vi "Begin.vi"() -> (0 "error out":errorcluster)   [LabVIEW 2013]
doc: "Called before other user functions, this VI is expected to open initial I/O refnums, load in file data, and do all program initialization. Notice that the <B>error out</B> terminal is simply used for data flow. Wiring it to other structures or subVIs ensures that this VI runs first."
uses:
  <vilib>/Rock Robotics/WPI/DriverStation/WPI_DriverStationRobotMode2.ctl
  <vilib>/Rock Robotics/WPI/Joystick/WPI_JoystickDeviceEnum.ctl
  <vilib>/Rock Robotics/SystemInterfaces/DIO/FPGA_DIOPWMChannel.ctl
  <vilib>/Rock Robotics/SystemInterfaces/Typedef/FPGA_TypedefDigitalModule.ctl
  <vilib>/Rock Robotics/WPI/SafetyOutput/WPI_SafetyOutputConfigMenu.ctl
  Robot Global Data.vi
  Device Refrences.vi
  <vilib>/Rock Robotics/WPI/RobotDrive/WPI_RobotDriveOpen2MotorWithJaguar.vi
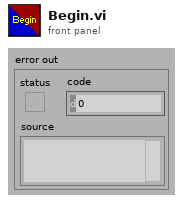
[diagram p1: front panel]
types:
  T1 = typedef "WPI_JoystickDeviceEnum.ctl" = enum16{"USB 1", "USB 2", "USB 3", "USB 4", "Kinect 1", "Kinect 2"}
  T2 = enum16{"1 3-axis Joystick", "2 2-axis Joysticks"}
  T3 = typedef "WPI_DriverStationRobotMode2.ctl" = enum16{"Autonomous Disabled", "Autonomous Enabled", "Teleop Disabled", "Teleop Enabled", "Timeout", "Finish", "Test Disabled", "Test Enabled"}
  T4 = typedef "WPI_JoystickDevRef.ctl" = cluster{"Device":T1}
  T5 = enum16{"Simulator Robot", "Alpinista", "2014 Robot"}
  T6 = typedef "FPGA_TypedefDigitalModule.ctl" = enum16{"Digital Module 1", "Digital Module 2"}
  T7 = typedef "FPGA_DIOPWMChannel.ctl" = enum8{"PWM 1", "PWM 2", "PWM 3", "PWM 4", "PWM 5", "PWM 6", "PWM 7", "PWM 8", "PWM 9", "PWM 10", "Invalid"}
  T8 = typedef "WPI_ServoDeviceRef.ctl" = cluster{"DeviceStatus":errorcluster, "Digital Module":T6, "PWM Channel":T7, "DeadBand":T9}
  T9 = typedef "WPI_PWMDeadband.ctl" = cluster{"Name":string, "maxPositivePwm":i32, "minPositivePwm":i32, "centerPwm":i32, "maxNegativePwm":i32, "minNegativePwm":i32, "angularRange":u16}
  T10 = typedef "WPI_SafetyOutputConfigMenu.ctl" = enum16{"Enable", "Disable"}
  T11 = typedef "WPI_RobotDriveDevRef.ctl" = cluster{"DevStatus":errorcluster, "Motors[]":T12[], "Square Inputs":bool, "Max Output":dbl, "Isochronous":bool}
  T12 = typedef "WPI_MotorControlDeviceRef.ctl" = cluster{"DeviceStatus":errorcluster, "Type":enum16{"PWM", "CAN"}, "PWM":cluster{"Digital Module":T6, "PWM Channel":T7, "DeadBand":T9}, "CAN":cluster{"Device Number":u8, "Control Mode":T13, "Semaphore":T14, "Max Vout":dbl}, "Invert":bool, "TransformRef":T15, "InvTransformRef":T15}
  T13 = typedef "WPI_CANJaguar_ControlMode.ctl" = enum8{"Percent VBus", "Current", "Speed", "Position", "Voltage"}
  T14 = typedef "Semaphore RefNum" = refnum<k1>
  T15 = typedef "WPI_PWMTransform_ConPane.ctl" = refnum<vi>
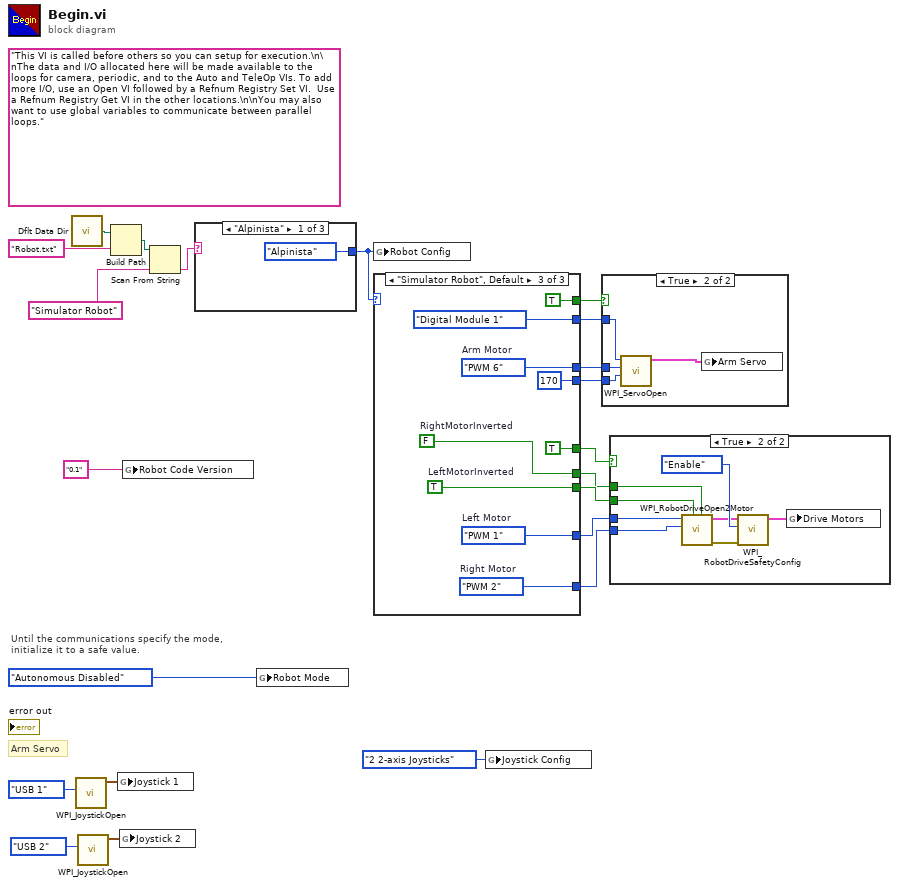
[diagram p0: block diagram]
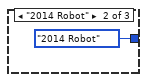
[diagram p4: hidden frame]
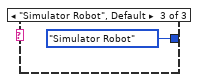
[diagram p5: hidden frame]
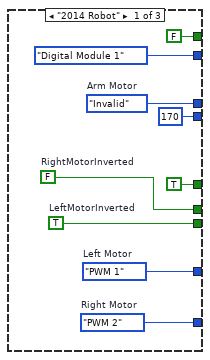
[diagram p6: hidden frame]
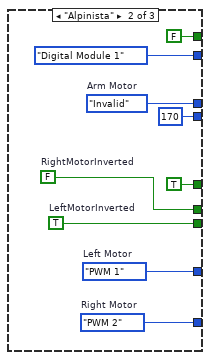
[diagram p7: hidden frame]
diagram:
  (unwired) "This VI is called before others so you can setup for execution.\n\nThe data and I/O allocated here will be made available to the loops for camera, periodic, and to the Auto and TeleOp VIs. To add more I/O, use an Open VI followed by a Refnum Registry Set VI.  Use a Refnum Registry Get VI in the other locations.\n\nYou may also want to use global variables to communicate between parallel loops."
  # "Arm Servo"
  # "Until the communications specify the mode,\ninitialize it to a safe value."
  n1 = call <vilib>:"Dflt Data Dir.vi"() -> ("App:Default Data Directory"=w11:path)
  n2 = call <vilib>:"WPI_JoystickOpen.vi"("JoystickDevice"=WPI_JoystickDeviceEnum."USB 1") -> ("JoystickDevRef"=w20:T4)  [unwired: 10 in]
  n3 = call <vilib>:"WPI_JoystickOpen.vi"("JoystickDevice"=WPI_JoystickDeviceEnum."USB 2") -> ("JoystickDevRef"=w2:T4)  [unwired: 10 in]
  n4 = Build Path(base path=w11, name or relative path="Robot.txt") -> (appended path=w5:path)
  n5 = global write "Device Refrences.vi" "Joystick 1"(w20) -> ()
  n6 = global write "Device Refrences.vi" "Joystick 2"(w2) -> ()
  n7 = global write "Robot Global Data.vi" "Robot Code Version"("0.1") -> ()
  n8 = Scan From String(w5, default 1="Simulator Robot") -> (output 1=w7:string)  [unwired: 2 in, 2 out]
  n9 = case shown="\"Alpinista\"" w7 {
    tunnel: [T5."Alpinista" ("Robot Config") T5."2014 Robot" ("Robot Config") T5."Simulator Robot" ("Robot Config")] -> w12
    frame "Alpinista" {
    }
    frame "2014 Robot" {
    }
    frame "Simulator Robot", Default {
    }
  }
  n10 = global write "Robot Global Data.vi" "Robot Mode"(WPI_DriverStationRobotMode2."Autonomous Disabled" ("Robot Mode")) -> ()
  n11 = global write "Robot Global Data.vi" "Robot Config"(w12) -> ()
  n12 = case shown="\"Simulator Robot\", Default" w12 {
    tunnel: [w28 w37 w52] -> w19
    tunnel: [w30 w39 w51] -> w18
    tunnel: [w31 w40 w50] -> w17
    tunnel: [w29 w38 w49] -> w16
    tunnel: [FPGA_TypedefDigitalModule."Digital Module 1" ("Digital Module (Module 1)") FPGA_TypedefDigitalModule."Digital Module 1" ("Digital Module (Module 1)") FPGA_TypedefDigitalModule."Digital Module 1" ("Digital Module (Module 1)")] -> w15
    tunnel: [w33 w43 w47] -> w14
    tunnel: [170 170 170] -> w13
    tunnel: [TRUE TRUE TRUE] -> w9
    tunnel: [FALSE FALSE TRUE] -> w8
    frame "2014 Robot" {
      w33 = FPGA_DIOPWMChannel."Invalid"  # Arm Motor
      w31 = FALSE  # RightMotorInverted
      w30 = TRUE  # LeftMotorInverted
      w28 = FPGA_DIOPWMChannel."PWM 2"  # Right Motor
      w29 = FPGA_DIOPWMChannel."PWM 1"  # Left Motor
    }
    frame "Alpinista" {
      w43 = FPGA_DIOPWMChannel."Invalid"  # Arm Motor
      w40 = FALSE  # RightMotorInverted
      w39 = TRUE  # LeftMotorInverted
      w37 = FPGA_DIOPWMChannel."PWM 2"  # Right Motor
      w38 = FPGA_DIOPWMChannel."PWM 1"  # Left Motor
    }
    frame "Simulator Robot", Default {
      w47 = FPGA_DIOPWMChannel."PWM 6"  # Arm Motor
      w50 = FALSE  # RightMotorInverted
      w51 = TRUE  # LeftMotorInverted
      w52 = FPGA_DIOPWMChannel."PWM 2"  # Right Motor
      w49 = FPGA_DIOPWMChannel."PWM 1"  # Left Motor
    }
  }
  n13 = global write "Robot Global Data.vi" "Joystick Config"(T2."2 2-axis Joysticks" ("Joystick Config")) -> ()
  n14 = case shown="True" w8 {
    tunnel: w15 -> [_ w55]
    tunnel: w14 -> [_ w54]
    tunnel: w13 -> [_ w53]
    frame False {
    }
    frame True {
      n15 = call <vilib>:"WPI_ServoOpen.vi"("Angular Range"=w53, "PWM Channel"=w54, "Digital Module (Module 1)"=w55) -> ("ServoDeviceRef"=w56:T8)  [unwired: 7 in, 1 out]
      n16 = global write "Device Refrences.vi" "Arm Servo"(w56) -> ()
    }
  }
  n17 = case shown="True" w9 {
    tunnel: w19 -> [_ w60]
    tunnel: w18 -> [_ w59]
    tunnel: w17 -> [_ w58]
    tunnel: w16 -> [_ w57]
    frame False {
    }
    frame True {
      n18 = call-poly <vilib>:"WPI_RobotDriveOpen2Motor.vi"("Right Motor Inverted"=w58, "Left Motor Inverted"=w59, "Right Motor"=w60, "Left Motor"=w57) -> ("error out"=w62:errorcluster, "RobotDriveDevRef"=w63:T11)  [unwired: 1 in, 5 out]
      n19 = call <vilib>:"WPI_RobotDriveSafetyConfig.vi"("error in (no error)"=w62, "mode"=WPI_SafetyOutputConfigMenu."Enable", "RobotDriveDevRef"=w63) -> ("RobotDriveDevRef"=w61:T11)  [unwired: 7 in, 1 out]
      n20 = global write "Device Refrences.vi" "Drive Motors"(w61) -> ()
    }
  }
